vi "wmf_properties.vi"() -> (2 "WMF Properties":string[](array[string])=["BRIGHTNESS", "CONTRAST", "HUE", "SATURATION", "SHARPNESS", "GAMMA", "COLORENABLE", "WHITEBALANCE", "BACKLIGHTCOMPENSATION", "GAIN", "PAN", "TILT", "ROLL", "ZOOM", "EXPOSURE", "IRIS", "FOCUS"])   [LabVIEW 2023, in "Vision.lvlib"]
uses:
  Vision.lvlib
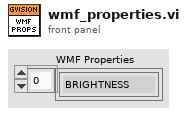
[diagram p1: front panel]
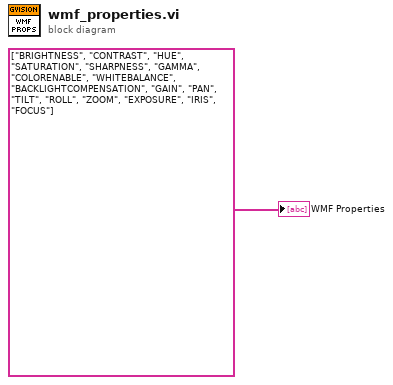
[diagram p0: block diagram]
diagram:
  "WMF Properties" <- string[] ["BRIGHTNESS", "CONTRAST", "HUE", "SATURATION", "SHARPNESS", "GAMMA", "COLORENABLE", "WHITEBALANCE", "BACKLIGHTCOMPENSATION", "GAIN", "PAN", "TILT", "ROLL", "ZOOM", "EXPOSURE", "IRIS", "FOCUS"]
